vi "Pre-Build Action.vi"() -> ()   [LabVIEW 2013]
uses:
  <vilib>/Utility/sysdir.llb/System Directory Type.ctl
panel:
  out "appended path":path
  out "data":string
  out "error out":errorcluster
  out "Tag:Get Names":string[](array[string])
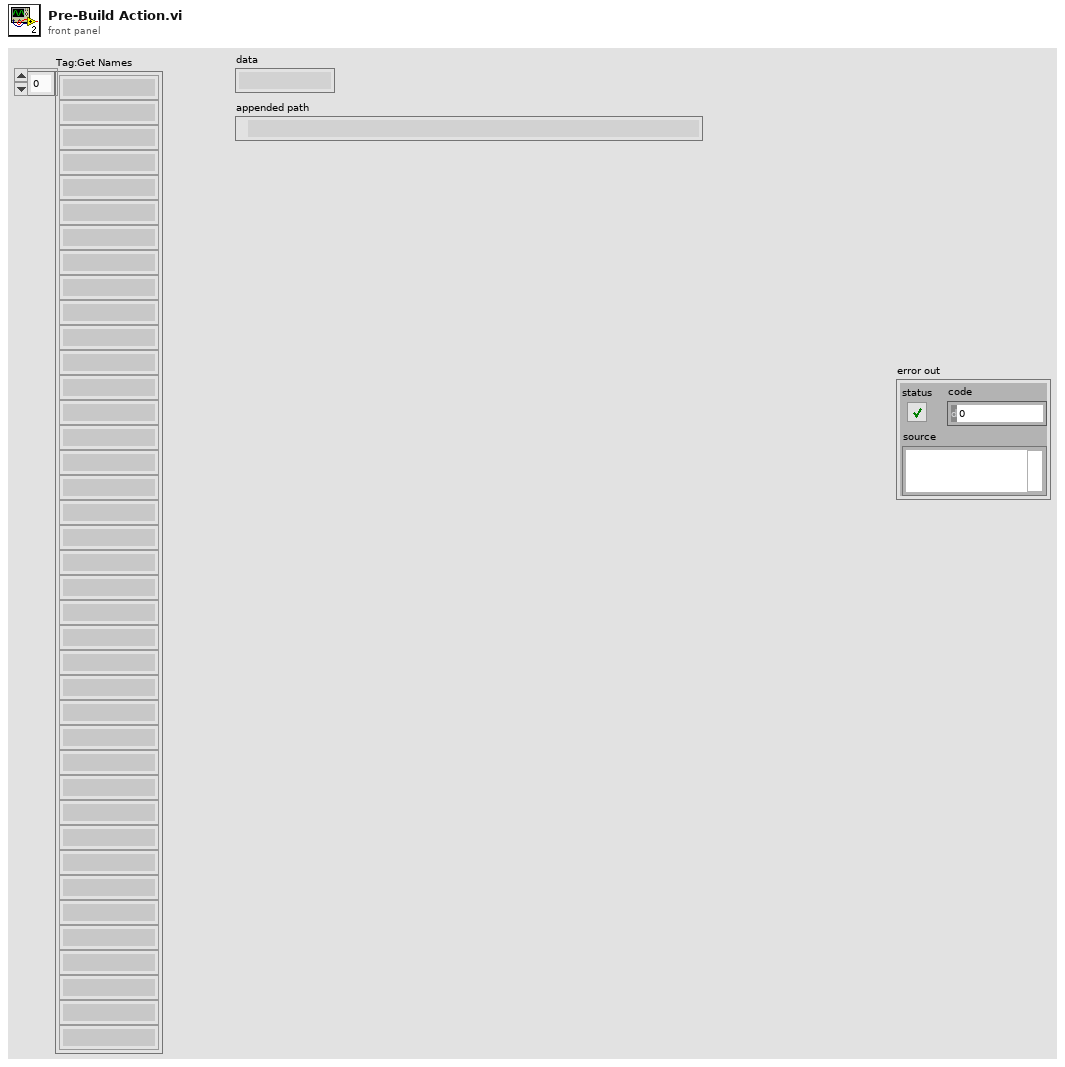
[diagram p1: front panel]
types:
  T1 = typedef "System Directory Type.ctl" = i32
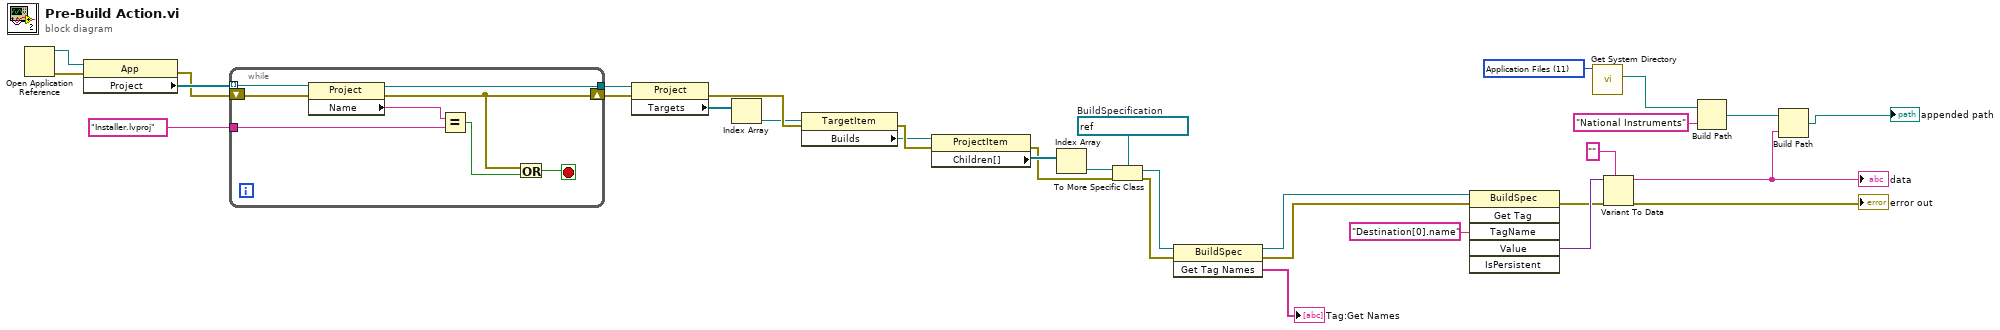
[diagram p0: block diagram]
diagram:
  w6 = T1 11 items=["User Home"=0, "User Desktop"=1, "User Documents"=2, "User Application Data"=3, "User Preferences"=4, "User Temporary"=5, "Public Documents"=6, "Public Application Data"=7, "Public Preferences"=8, "Public Cache"=13, "System Core Libraries"=9, "System Installed Libraries"=10, "Application Files"=11, "Boot Volume Root"=12] ("system directory type")
  w18 = refnum<vi> refnum  # BuildSpecification
  n1 = Open Application Reference() -> (0:w28:errorcluster, 3:w32:refnum<vi>)  [unwired: 4 in]
  n2 = property class="App"(reference=w32, error in=w28) -> (error out=w29:errorcluster, "Project"=w31:refnum<vi>[])  [unwired: 1 out]
  n3 = while {
    tunnel: w31 -> [w40] mode=indexing
    tunnel: "Installer.lvproj" -> [w38]
    tunnel: [w37] -> w26
    shift-right: [w34] -> w27
    shift-left: w29 -> [w36]
    stop <- w33 stop-if-true
    n4 = property class="Project"(reference=w40, error in=w36) -> (reference out=w37:refnum<vi>, error out=w34:errorcluster, "Name"=w39:string)
    n5 = Equal?(x=w39, y=w38) -> (x = y?=w35:bool)
    n6 = Or(x=w34, y=w35) -> (x .or. y?=w33:bool)
  }
  n7 = property class="Project"(reference=w26, error in=w27) -> (error out=w24:errorcluster, "Targets"=w25:refnum<vi>[])  [unwired: 1 out]
  n8 = Index Array(array=w25) -> (element=w23:refnum<vi>)  [unwired: 1 in]
  n9 = property class="TargetItem"(reference=w23, error in=w24) -> (error out=w22:errorcluster, "Builds"=w21:refnum<vi>)  [unwired: 1 out]
  n10 = property class="ProjectItem"(reference=w21, error in=w22) -> (error out=w14:errorcluster, "Children[]"=w20:refnum<vi>[])  [unwired: 1 out]
  n11 = Index Array(array=w20) -> (element=w19:refnum<vi>)  [unwired: 1 in]
  n12 = To More Specific Class(target class=w18, reference=w19, error in=w14) -> (specific class reference=w17:refnum<vi>, error out=w13:errorcluster)
  n13 = invoke class="BuildSpec" method="Get Tag Names"(reference=w17, error in=w13) -> (reference out=w15:refnum<vi>, error out=w12:errorcluster, "Get Tag Names"=→"Tag:Get Names":string[])  [unwired: 1 in]
  n14 = invoke class="BuildSpec" method="Get Tag"(reference=w15, error in=w12, "TagName"="Destination[0].name" ("Tag Name")) -> (error out=w9:errorcluster, "Value"=w10:variant)  [unwired: 3 in, 4 out]
  n15 = call <vilib>:"Get System Directory.vi"("system directory type"=w6) -> ("system directory"=w5:path)  [unwired: 10 in]
  n16 = Variant To Data(error in=w9, type="", Variant=w10) -> (data=w2:string, error out=→"error out":errorcluster)
  "data" <- w2
  n17 = Build Path(base path=w5, name or relative path="National Instruments") -> (appended path=w3:path)
  n18 = Build Path(base path=w3, name or relative path=w2) -> (appended path=→"appended path":path)
